vi "EX_OR.vi"() -> ()   [LabVIEW 2024]
panel:
  in  "y":bool
  in  "x":bool
  out "x .or. y?":bool
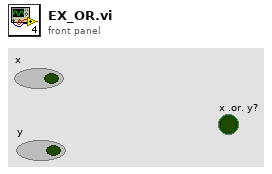
[diagram p1: front panel]
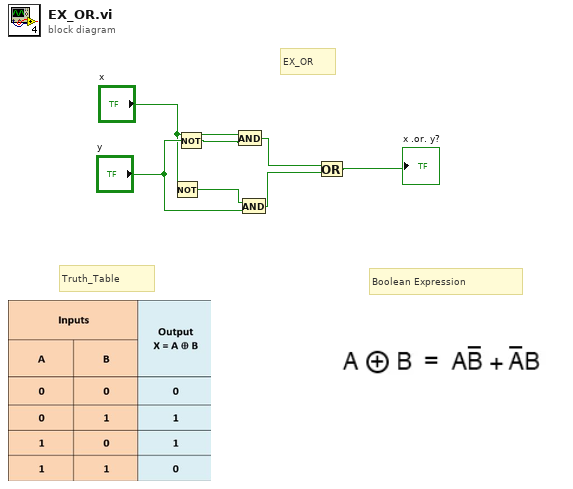
[diagram p0: block diagram]
diagram:
  # "EX_OR"
  # "Truth_Table"
  # "Boolean Expression"
  n1 = Not(x="x") -> (.not. x?=w7:bool)
  n2 = Not(x="y") -> (.not. x?=w5:bool)
  n3 = And(x="x", y=w5) -> (x .and. y?=w3:bool)
  n4 = And(x=w7, y="y") -> (x .and. y?=w2:bool)
  n5 = Or(x=w3, y=w2) -> (x .or. y?=→"x .or. y?":bool)
